vi "edittest build ALLDATASHEETS object.vi"(7 "Template (empty)":T1, 8 "error in (no error)":errorcluster, 11 "Connection Refnum":T2) -> (0 "error out":errorcluster, 3 "Connection Refnum":T2, 5 "new Template":T1)   [LabVIEW 2011]
uses:
  SI.LIB/ODBC/SQL Controls/Connection Refnum.ctl
  Addons/internet/utils/keyedarr.llb/Keyed Array.ctl
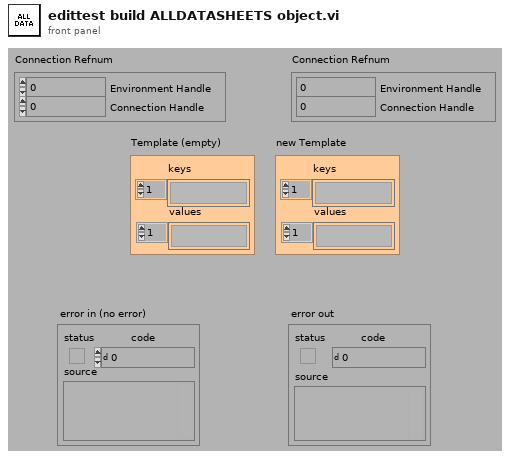
[diagram p1: front panel]
types:
  T1 = typedef "Keyed Array.ctl" = cluster{"keys":string[], "values":string[]}
  T2 = typedef "Connection Refnum.ctl" = cluster{"Environment Handle":i32, "Connection Handle":i32}
  T3 = typedef "Template Record.ctl" = cluster{"ixTemplate":i32, "sxTemplateId":string, "sDescription":string, "sCreator":string, "tCreationDate":timestamp, "sModifier":string, "tModifiedDate":timestamp, "sType":string, "sStyle":string, "sFormat":string, "dWidth":dbl, "dHeight":dbl, "sFilename":string, "sScript":string, "sLayout":string, "sEditor":string, "sStyleProcess":string}
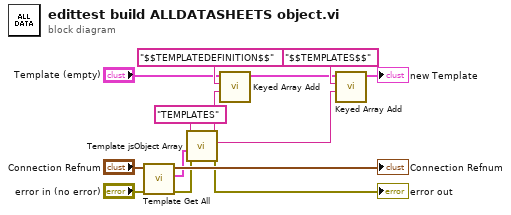
[diagram p0: block diagram]
diagram:
  n1 = call "Template Get All.vi"("error in (no error)"="error in (no error)", "Connection Refnum"="Connection Refnum") -> ("error out"=w9:errorcluster, "Templates"=w11:T3[], "Connection Refnum"=→"Connection Refnum":T2)  [unwired: 1 in, 6 out]
  n2 = call "Template jsObject Array.vi"("error in (no error)"=w9, "TEMPLATES (none)"=w11, "Array Name (\"TEMPLATES\")"="TEMPLATES" ("Array Name (\"\")")) -> ("error out"=→"error out":errorcluster, "Templates jsObject Array"=w3:string, "Template jsObject Definition"=w4:string)  [unwired: 1 in, 5 out]
  n3 = call "Keyed Array Add.vi"("value"=w4, "key"="$$TEMPLATEDEFINITION$$" ("Array Name (\"\")"), "array in"="Template (empty)") -> ("array out"=w1:T1)  [unwired: 1 in, 3 out]
  n4 = call "Keyed Array Add.vi"("value"=w3, "key"="$$TEMPLATES$$" ("Array Name (\"\")"), "array in"=w1) -> ("array out"=→"new Template":T1)  [unwired: 1 in, 3 out]
